vi "Get Dynamical System.vi"(8 "dt":dbl, 11 "Dynamical System":T2) -> (2 "G (Control Input Matrix)":T1, 3 "F (State Transition Matrix)":T1)   [LabVIEW 2020]
uses:
  ctl/Dynamical System Templates.ctl
  <vilib>/Analysis/Matrix/Datatypes/RealMatrix.ctl
  <vilib>/Analysis/Matrix/NI_Matrix.lvlib
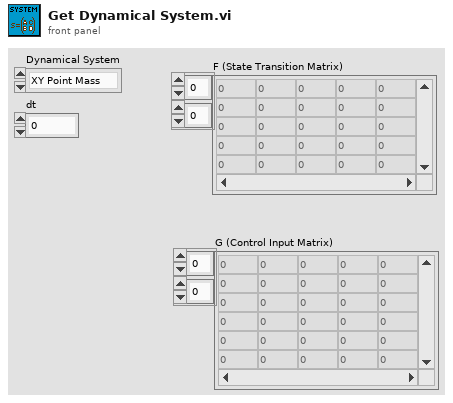
[diagram p1: front panel]
types:
  T1 = typedef "NI_Matrix.lvlib/RealMatrix.ctl" = dbl[][]
  T2 = typedef "Dynamical System Templates.ctl" = enum16{"XY Point Mass"}
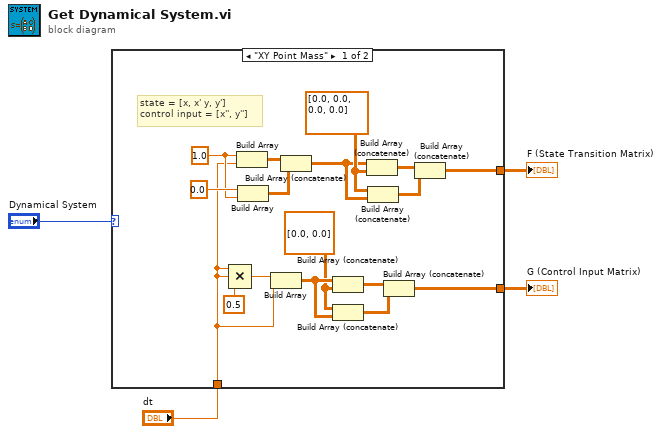
[diagram p0: block diagram]
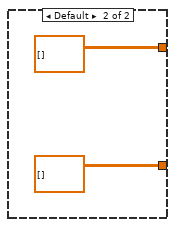
[diagram p2: hidden frame]
diagram:
  n1 = case shown="\"XY Point Mass\"" "Dynamical System" {
    tunnel: [w12 T1 [] ("matrix")] -> w2
    tunnel: [w5 T1 [] ("matrix")] -> w1
    tunnel: "dt" -> [w10 _]
    frame "XY Point Mass" {
      w8 = T1 [[0.0], [0.0]] ("matrix")
      w16 = T1 [[0.0, 0.0], [0.0, 0.0]] ("matrix")
      w19 = 1.0 ("element")
      # "state = [x, x' y, y']\ncontrol input = [x'', y'']"
      n2 = Compound Arithmetic op=MULTIPLY(w10, w10, 0.5 ("value")) -> (w11:dbl)
      n3 = Build Array(w19, w10) -> (w17:T1)
      n4 = Build Array(0.0 ("element"), w19) -> (w18:T1)
      n5 = Build Array(w11, w10) -> (w9:T1)
      n6 = Build Array (concatenate)(w17, w18) -> (w15:T1)
      n7 = Build Array (concatenate)(w9, w8) -> (w7:T1)
      n8 = Build Array (concatenate)(w8, w9) -> (w6:T1)
      n9 = Build Array (concatenate)(w15, w16) -> (w14:T1)
      n10 = Build Array (concatenate)(w16, w15) -> (w13:T1)
      n11 = Build Array (concatenate)(w7, w6) -> (w5:T1)
      n12 = Build Array (concatenate)(w14, w13) -> (w12:T1)
    }
    frame Default {
    }
  }
  "F (State Transition Matrix)" <- w2
  "G (Control Input Matrix)" <- w1
